vi "Take Snapshot.vi"(8 "error in":errorcluster, 11 "AnalogInput in":refnum<class "AnalogInput.lvclass">) -> (0 "error out":errorcluster, 3 "AnalogInput out":refnum<class "AnalogInput.lvclass">)   [LabVIEW 2019, in "AnalogInput.lvlib" / "AnalogInput.lvclass"]
doc: "Use Snapshot Data to Generate a Group Separated Snapshot record. This eliminates nearly all the overhead in creating and removing a record group for snapshot data."
uses:
  Library/AnalogInput.lvclass
  C:/Users/Public/Documents/Development/builds/Instruments/Instruments.lvlibp/Library/Instruments.lvclass
  Library/AnalogInput.lvclass/AnalogInput.ctl
  Accessors/Triggering/Read Trigger Source.vi
  Accessors/Triggering/Read Trigger Settings.vi
  builds/Instruments/Instruments.lvlibp/Private/Polymorphic/Special/Event from String.vi
  builds/Instruments/Instruments.lvlibp/Accessors/Command with Logging.vi
  builds/Instruments/Instruments.lvlibp/Library/Instruments.lvclass
  builds/Instruments/Instruments.lvlibp
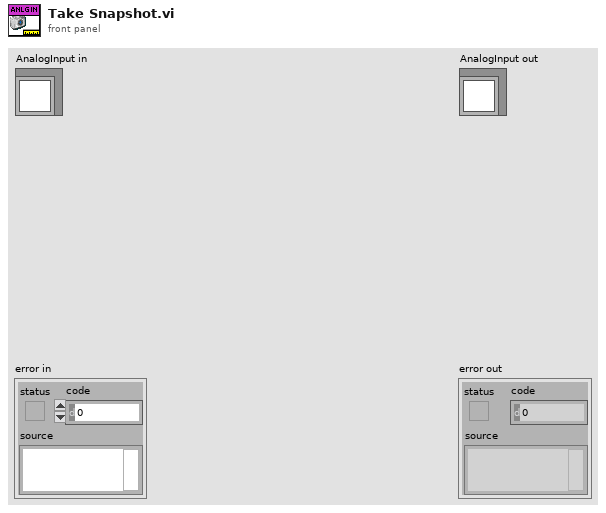
[diagram p1: front panel]
types:
  T1 = typedef "AnalogInput.lvlib/AnalogInput.lvclass/User Trigger Settings.ctl" = cluster{"Timeout":dbl, "Level":dbl, "Slope":T2, "samples per channel":i32, "Sample Rate (10k)":dbl, "pretrigger samples":u32}
  T2 = typedef "AnalogInput.lvlib/AnalogInput.lvclass/Trigger_Slope.ctl" = enum16{"Rising", "Falling"}
  T3 = cluster{"Timestamp":timestamp, "Description":string, "Data":string}
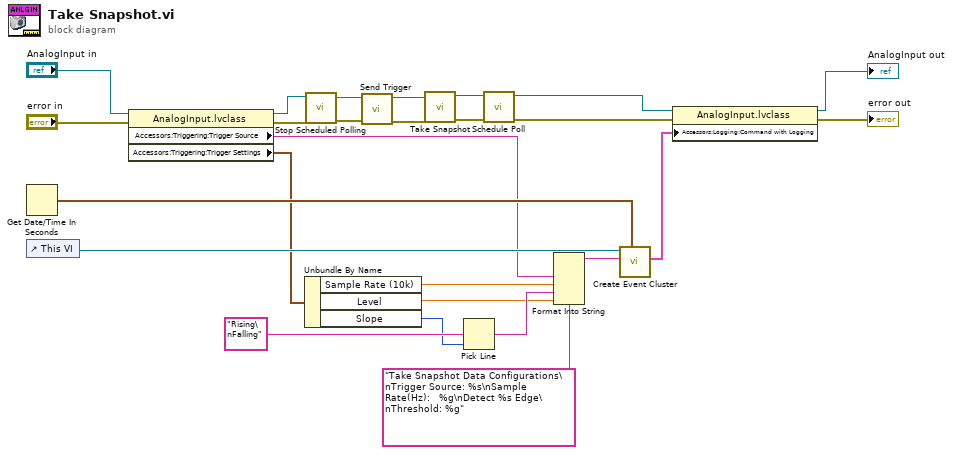
[diagram p0: block diagram]
diagram:
  n1 = Get Date/Time In Seconds() -> (seconds since 1Jan1904=w9:timestamp)
  n2 = control-ref of="This VI"() -> (w16:refnum<vi>)
  n3 = property class="AnalogInput.lvclass"(reference="AnalogInput in", error in="error in") -> (reference out=w12:refnum<class "AnalogInput.lvclass">, error out=w11:errorcluster, "Accessors:Triggering:Trigger Source"=w2:string, "Accessors:Triggering:Trigger Settings"=w1:T1)
  n4 = Unbundle By Name(w1) -> ("Sample Rate (10k)"=w7:dbl, "Level"=w4:dbl, "Slope"=w3:T2)
  n5 = call "Stop Scheduled Polling.vi"("error in"=w11, "Instruments in"=w12) -> ("error out"=w23:errorcluster, "Instruments out"=w24:refnum<class "AnalogInput.lvclass">)  [unwired: 8 in]
  n6 = call-dynamic "Send Trigger.vi"("error in (no error)"=w23, "AnalogInput in"=w24) -> ("error out"=w22:errorcluster, "AnalogInput out"=w21:refnum<class "AnalogInput.lvclass">)  [unwired: 8 in]
  n7 = call-parent "Take Snapshot.vi"("error in"=w22, "Instruments in"=w21) -> ("error out"=w25:errorcluster, "Instruments out"=w26:refnum<class "AnalogInput.lvclass">)  [unwired: 8 in]
  n8 = Pick Line(multi-line string="Rising\nFalling", line index=w3) -> (output string=w5:string)  [unwired: 1 in]
  n9 = call "Schedule Poll.vi"("error in"=w25, "Instruments in"=w26) -> ("error out"=w19:errorcluster, "Instruments out"=w20:refnum<class "AnalogInput.lvclass">)  [unwired: 8 in]
  n10 = Format Into String(format string="Take Snapshot Data Configurations\nTrigger Source: %s\nSample Rate(Hz):   %g\nDetect %s Edge\nThreshold: %g", w2, w7, w5, w4) -> (resulting string=w10:string)  [unwired: 2 in, 1 out]
  n11 = call-poly "Create Event Cluster.vi"("Time Stamp"=w9, "Value"=w10, "VI Refnum"=w16) -> ("Event Data"=w15:T3)  [unwired: 8 in]
  n12 = property class="AnalogInput.lvclass"(reference=w20, error in=w19, "Accessors:Logging:Command with Logging"=w15) -> (reference out=→"AnalogInput out":refnum<class "AnalogInput.lvclass">, error out=→"error out":errorcluster)
